vi "Handle Message.vi"(8 "error in (no error)":errorcluster, 11 "OOQMH in":refnum<class "OOQMH.lvclass">) -> (0 "error out":errorcluster, 3 "OOQMH out":refnum<class "OOQMH.lvclass">)   [LabVIEW 2024, in "OOQMH.lvlib" / "OOQMH.lvclass"]
uses:
  OOQMH.lvclass
  OOQMH.lvclass/OOQMH.ctl
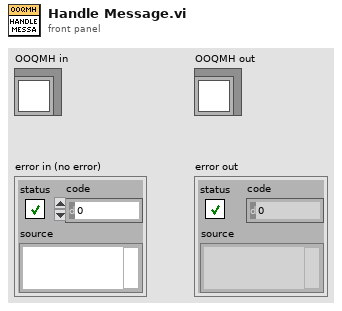
[diagram p1: front panel]
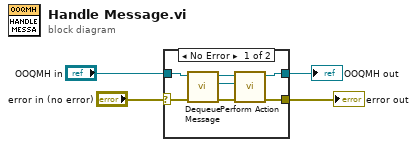
[diagram p0: block diagram]
diagram:
  n1 = case shown="No Error" "error in (no error)" {
    selector: "error in (no error)" -> [w8 w13]
    tunnel: [w10 w13] -> w3
    tunnel: [w11 w12] -> w1
    tunnel: "OOQMH in" -> [w9 w12]
    frame No Error {
      n2 = call-dynamic "Dequeue Message.vi"("error in (no error)"=w8, "OOQMH in"=w9) -> ("error out"=w5:errorcluster, "Message out"=w6:refnum<class "Message.lvclass">, "OOQMH out"=w7:refnum<class "OOQMH.lvclass">)  [unwired: 7 in]
      n3 = call-dynamic "Perform Action.vi"("error in (no error)"=w5, "Message in"=w6, "OOQMH in"=w7) -> ("error out"=w10:errorcluster, "OOQMH out"=w11:refnum<class "OOQMH.lvclass">)  [unwired: 7 in]
    }
    frame Error {
    }
  }
  "error out" <- w3
  "OOQMH out" <- w1
